vi "Alignment.vi"(0 "Sensor":enum16{"Ultrasonic", "Camera", "Gyro"}(ring)) -> ()   [LabVIEW 2013]
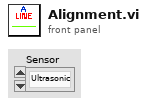
[diagram p1: front panel]
types:
  T1 = typedef "TargetType.ctl" = enum16{"Not Hot", "Hot"}
  T2 = cluster{"Scores":cluster{"Total":dbl, "Left":dbl, "Right":dbl, "Ratio":dbl, "Vertical":dbl, "index":i32, "State":T1}, "Verticals":cluster{"Horizontal?":bool, "Aspect Score":dbl, "Rect Score":dbl, cluster{"Left":dbl, "Top":dbl, "Right":dbl, "Bottom":dbl}, "Equiv H":dbl, "Equiv V":dbl}, "Horizontals":cluster{"Horizontal?":bool, "Aspect Score":dbl, "Rect Score":dbl, cluster{"Left":dbl, "Top":dbl, "Right":dbl, "Bottom":dbl}, "Equiv H":dbl, "Equiv V":dbl}, "Distance ft":dbl, "Center":cluster{"X":dbl, "Y":dbl}}[]
  T3 = cluster{"Scores":cluster{"Total":dbl, "Left":dbl, "Right":dbl, "Ratio":dbl, "Vertical":dbl, "index":i32, "State":T1}, "Verticals":cluster{"Horizontal?":bool, "Aspect Score":dbl, "Rect Score":dbl, cluster{"Left":dbl, "Top":dbl, "Right":dbl, "Bottom":dbl}, "Equiv H":dbl, "Equiv V":dbl}, "Horizontals":cluster{"Horizontal?":bool, "Aspect Score":dbl, "Rect Score":dbl, cluster{"Left":dbl, "Top":dbl, "Right":dbl, "Bottom":dbl}, "Equiv H":dbl, "Equiv V":dbl}, "Distance ft":dbl, "Center":cluster{"X":dbl, "Y":dbl}}
  T4 = cluster{"Horizontal?":bool, "Aspect Score":dbl, "Rect Score":dbl, cluster{"Left":dbl, "Top":dbl, "Right":dbl, "Bottom":dbl}, "Equiv H":dbl, "Equiv V":dbl}
  T5 = cluster{"Left":dbl, "Top":dbl, "Right":dbl, "Bottom":dbl}
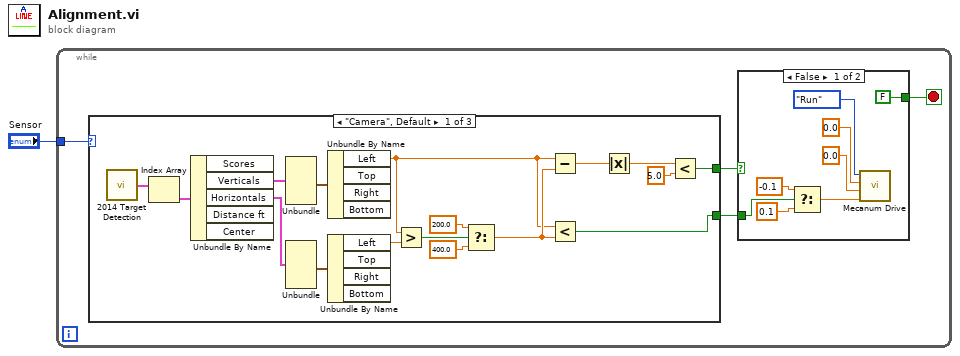
[diagram p0: block diagram]
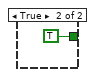
[diagram p2: hidden frame]
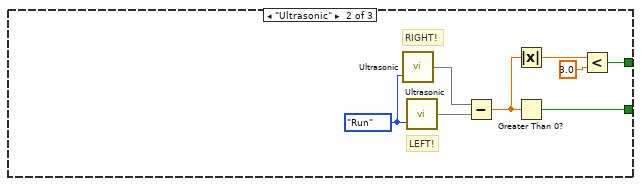
[diagram p3: hidden frame]
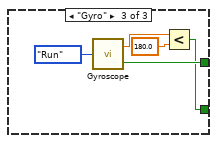
[diagram p4: hidden frame]
diagram:
  n1 = while {
    tunnel: "Sensor" -> [w5]
    stop <- w2 stop-if-true
    n2 = case shown="\"Camera\", Default" w5 {
      tunnel: [w15 w32 w40] -> w3
      tunnel: [w16 w34 w41] -> w4
      frame "Camera", Default {
        n3 = call "2014 Target Detection.vi"() -> ("Target Info"=w25:T2)  [unwired: 1 in]
        n4 = Index Array(array=w25) -> (element=w24:T3)  [unwired: 1 in]
        n5 = Unbundle By Name(w24) -> ("Verticals"=w23:T4, "Horizontals"=w22:T4)  [unwired: 3 out]
        n6 = Unbundle(w23) -> (w21:T5)  [unwired: 5 out]
        n7 = Unbundle(w22) -> (w20:T5)  [unwired: 5 out]
        n8 = Unbundle By Name(w21) -> ("Left"=w17:dbl)  [unwired: 3 out]
        n9 = Unbundle By Name(w20) -> ("Left"=w19:dbl)  [unwired: 3 out]
        n10 = Greater?(x=w17, y=w19) -> (0:w28:bool)
        n11 = Select(t=200.0 ("y"), s=w28, f=400.0 ("y")) -> (s? t:f=w18:dbl)
        n12 = Subtract(x=w17, y=w18) -> (x-y=w31:dbl)
        n13 = Less?(x=w17, y=w18) -> (x < y?=w15:bool)
        n14 = Absolute Value(x=w31) -> (abs(x)=w30:dbl)
        n15 = Less?(x=w30, y=5.0) -> (x < y?=w16:bool)
      }
      frame "Ultrasonic" {
        w37 = enum16{"Open", "Run", "End"}."Run" ("State Control")
        # "LEFT!"
        # "RIGHT!"
        n16 = call "Ultrasonic.vi"("Right"=w37) -> (0:w36)  [unwired: 1 in]
        n17 = call "Ultrasonic.vi"("Right"=w37) -> (0:w35)  [unwired: 1 in]
        n18 = Subtract(x=w36, y=w35) -> (x-y=w33:dbl)
        n19 = Absolute Value(x=w33) -> (abs(x)=w39:dbl)
        n20 = Greater Than 0?(x=w33) -> (x > 0?=w32:bool)
        n21 = Less?(x=w39, y=3.0) -> (x < y?=w34:bool)
      }
      frame "Gyro" {
        n22 = call "Gyroscope.vi"("State Control"=enum16{"Open", "Run", "End"}."Run") -> ("Angle"=w42:dbl, "Initial Position?"=w41:bool)
        n23 = Less?(x=w42, y=180.0) -> (x < y?=w40:bool)
      }
    }
    n24 = case shown="False" w4 {
      tunnel: [FALSE TRUE] -> w2
      tunnel: w3 -> [w6 _]
      frame False {
        n25 = Select(t=-0.1 ("Turning"), s=w6, f=0.1 ("Turning")) -> (s? t:f=w8:dbl)
        n26 = call "Mecanum Drive.vi"("Turning"=w8, "F/R"=0.0, "Strafing"=0.0, "State Control"=enum16{"Open", "Run", "End"}."Run") -> ()
      }
      frame True {
      }
    }
  }
